vi "Execute In Python.vi"(0 "code":string, 5 "working directory":path, 11 "error in (no error)":errorcluster) -> (4 "stdout":string, 15 "error out":errorcluster)   [LabVIEW 2015, in "LV System Utils v1.lvlib"]
doc: "Executes code in python interpreter. Returns stdout.\nstderr becomes a message in the error cluster.\nReturn code becomes a code in the error cluster.\nIf return code is different than 0, status in error cluster becomes True.\nNote: 'python' command must be added to the PATH system variable."
uses:
  LV System Utils v1.lvlib
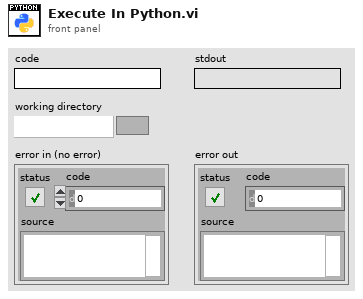
[diagram p1: front panel]
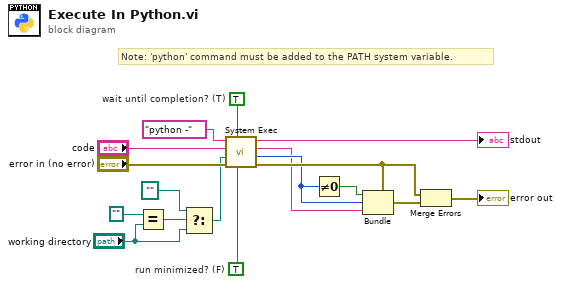
[diagram p0: block diagram]
diagram:
  w6 = TRUE  # run minimized? (F)
  w7 = TRUE  # wait until completion? (T)
  # "Note: 'python' command must be added to the PATH system variable."
  n1 = Equal?(x=path "", y="working directory") -> (x = y?=w5:bool)
  n2 = Select(t=path "" ("Application Directory"), s=w5, f="working directory") -> (s? t:f=w2:path)
  n3 = call <vilib>:"System Exec.vi"("run minimized? (F)"=w6, "wait until completion? (T)"=w7, "error in (no error)"="error in (no error)", "working directory"=w2, "standard input"="code", "command line"="python -") -> ("error out"=w13:errorcluster, "return code"=w10:i32, "standard error"=w9:string, "standard output"=→"stdout":string)  [unwired: 2 in]
  n4 = Not Equal To 0?(x=w10) -> (x != 0?=w11:bool)
  n5 = Bundle(cluster=w13, "status"=w11, "code"=w10, "source"=w9) -> (w12:errorcluster)
  n6 = Merge Errors(w13, w12) -> (→"error out":errorcluster)
